vi "Resize Private Data Panel.vi"(8 "error in (no error)":errorcluster, 11 "Private Data Refs":T1) -> (0 "error out":errorcluster)   [LabVIEW 2020, in "Add to Private Data.lvlib"]
uses:
  Add to Private Data.lvlib
  Private Data Refs.ctl
  <vilib>/Utility/miscctls.llb/LVPointTypeDef.ctl
  <vilib>/Utility/miscctls.llb/LVPositionTypeDef.ctl
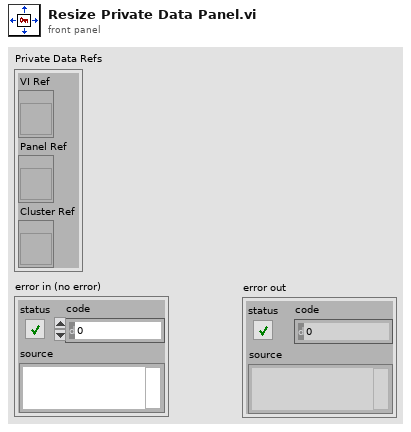
[diagram p1: front panel]
types:
  T1 = typedef "Add to Private Data.lvlib/Private Data Refs.ctl" = cluster{"VI Ref":refnum<vi>, "Panel Ref":refnum<vi>, "Cluster Ref":refnum<vi>}
  T2 = typedef "LVPositionTypeDef.ctl" = cluster{"Left":i32, "Top":i32}
  T3 = typedef "LVPointTypeDef.ctl" = cluster{"Horizontal":i16, "Vertical":i16}
  T4 = typedef "LVRectTypeDef.ctl" = cluster{"Left":i16, "Top":i16, "Right":i16, "Bottom":i16}
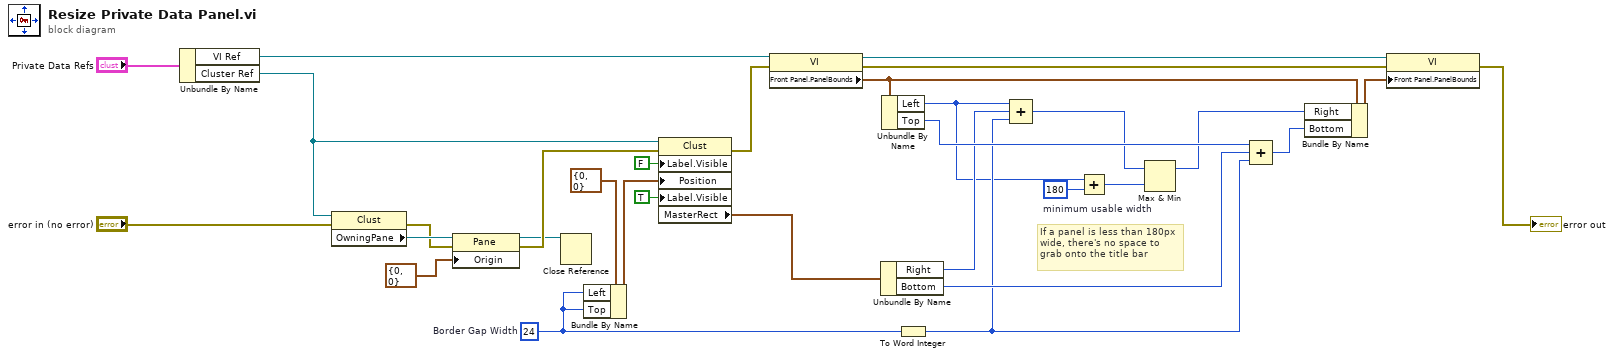
[diagram p0: block diagram]
diagram:
  w8 = i16 180  # minimum usable width
  w10 = 24  # Border Gap Width
  # "If a panel is less than 180px\nwide, there's no space to\ngrab onto the title bar"
  n1 = Unbundle By Name("Private Data Refs") -> ("VI Ref"=w2:refnum<vi>, "Cluster Ref"=w1:refnum<vi>)
  n2 = property class="Clust"(reference=w1, error in="error in (no error)") -> (error out=w24:errorcluster, "OwningPane"=w28:refnum<vi>)  [unwired: 1 out]
  n3 = property class="Pane"(reference=w28, error in=w24, "Origin"=T3 {"Horizontal"=0, "Vertical"=0}) -> (reference out=w20:refnum<vi>, error out=w25:errorcluster)
  n4 = Close Reference(reference=w20) -> ()  [unwired: 1 in, 1 out]
  n5 = Bundle By Name(cluster=T2 {"Left"=0, "Top"=0} ("Position"), "Left"=w10, "Top"=w10) -> (w14:T2)
  n6 = property class="Clust"(reference=w1, error in=w25, "Label.Visible"=FALSE, "Position"=w14, "Label.Visible"=TRUE) -> (error out=w13:errorcluster, "MasterRect"=w23:T4)  [unwired: 1 out]
  n7 = property class="VI"(reference=w2, error in=w13) -> (reference out=w21:refnum<vi>, error out=w12:errorcluster, "Front Panel.PanelBounds"=w19:T4)
  n8 = Unbundle By Name(w23) -> ("Right"=w18:i16, "Bottom"=w17:i16)
  n9 = Unbundle By Name(w19) -> ("Left"=w6:i16, "Top"=w31:i16)
  n10 = To Word Integer(number=w10) -> (16bit integer=w9:i16)
  n11 = Compound Arithmetic op=ADD(w6, w18, w9) -> (w5:i16)
  n12 = Add(x=w6, y=w8) -> (x+y=w7:i16)
  n13 = Max & Min(x=w5, y=w7) -> (max(x,y)=w4:i16)  [unwired: 1 out]
  n14 = Compound Arithmetic op=ADD(w31, w17, w9) -> (w16:i16)
  n15 = Bundle By Name(cluster=w19, "Right"=w4, "Bottom"=w16) -> (w22:T4)
  n16 = property class="VI"(reference=w21, error in=w12, "Front Panel.PanelBounds"=w22) -> (error out=→"error out":errorcluster)  [unwired: 1 out]
